vi "Release v1.0.vi"() -> ()   [LabVIEW 2014]
uses:
  <vilib>/Instr/_visa.llb/VISA Configure Serial Port (Instr).vi
  <vilib>/addons/control/pid/NI_PID_autopid.lvlib
panel:
  in  "Tab Control":T1(tab)
  in  "yaw PID gains":T2={"proportional gain (Kc)"=0.1, "integral time (Ti, min)"=0.001, "derivative time (Td, min)"=0.001} {"derivative time (Td, min)" step=0.001 format="%.3f"; "integral time (Ti, min)" step=0.01 format="%.3f"; "proportional gain (Kc)" step=0.1 format="%.3f"}
  in  "pitch PID gains":T2={"proportional gain (Kc)"=0.1, "integral time (Ti, min)"=0.001, "derivative time (Td, min)"=0.001} {"derivative time (Td, min)" step=0.001 format="%.3f"; "integral time (Ti, min)" step=0.01 format="%.3f"; "proportional gain (Kc)" step=0.1 format="%.3f"}
  in  "roll PID gains":T2={"proportional gain (Kc)"=0.1, "integral time (Ti, min)"=0.001, "derivative time (Td, min)"=0.001} {"derivative time (Td, min)" step=0.001 format="%.3f"; "integral time (Ti, min)" step=0.01 format="%.3f"; "proportional gain (Kc)" step=0.1 format="%.3f"}
  out "Celda 4":dbl
  out "Celda 3":dbl
  out "Celda 2":dbl
  out "Celda 1":dbl
  out "Celda 1":dbl(slide) scale=-1250.0..1250.0
  out "Celda 2":dbl(slide) scale=-1250.0..1250.0
  out "Celda 3":dbl(slide) scale=-1250.0..1250.0
  out "Celda 4":dbl(slide) scale=-1250.0..1250.0
  out "YAW PID":dbl
  out "yaw":cluster{"roll":dbl, "ROLL":dbl, dbl}(graph)
  out "yaw imu":dbl
  out "pitch imu":dbl
  out "PITCH PID":dbl
  out "PITCH":cluster{"roll":dbl, "ROLL":dbl, dbl}(graph)
  out "roll imu":dbl
  out "ROLL PID":dbl
  out "ROLL":cluster{"roll":dbl, "ROLL":dbl, dbl}(graph)
  out "Altura SENS":dbl
  in  "YAW":dbl(slide) scale=-25.0..25.0
  in  "PITCH 2":dbl(slide) caption="Roll" scale=-10.0..20.0
  in  "ROLL":dbl(slide) scale=-20.0..10.0
  in  "X":i64(slide) scale=-30.0..30.0
  in  "Y":i64(slide) scale=-30.0..30.0
  in  "?":i64(slide)=260 step=5 scale=220.0..290.0
  in  "PID ON?":bool
  out "bytes read":u32
  out "read string":string
  in  "stop":bool
  in  "baud rate":u32=115200
  in  "data bits":u16=8 min=5 max=8 step=1
  in  "parity":u16(ring) items=["None", "Odd", "Even", "Mark", "Space"]
  in  "stop bits":u16=10
  in  "flow control":u16
  in  "timeout (ms)":u32=10000
  in  "buffer size":u32=256
  in  "instr name":string="Arduino"
  in  "error in":errorcluster
  out "error out":errorcluster
  out "status":bool
  out "X 2":dbl
  out "Y 2":dbl
  out "Z":dbl
  in  "Stop":bool
  out "Write Buffer":string
  out "servo 2":dbl
  out "servo 4":dbl
  out "servo 5":dbl
  out "servo 6":dbl
  out "servo 1":dbl
  out "servo 3":dbl
  # "error"
  # "error"
  # "error"
  # "Z"
  # "el servo 1 responde al reves que los otros 5"
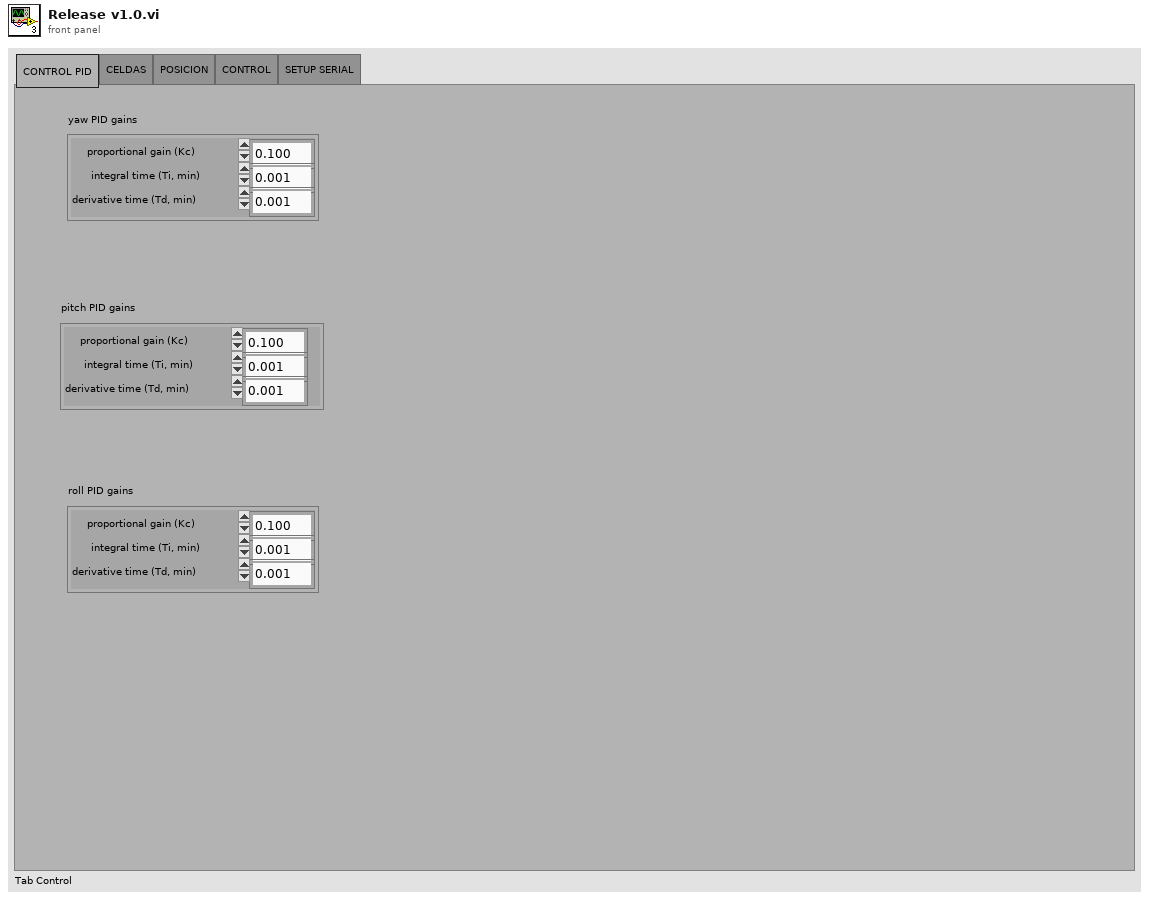
[diagram p1: front panel]
types:
  T1 = enum32{"CONTROL PID", "CELDAS", "POSICION", "CONTROL", "SETUP SERIAL"}
  T2 = cluster{"proportional gain (Kc)":dbl, "integral time (Ti, min)":dbl, "derivative time (Td, min)":dbl}
  T3 = cluster{"controller type":u16, "relay cycles":i32, "relay amplitude":dbl, "control specification":u16, "PV noise level":dbl}
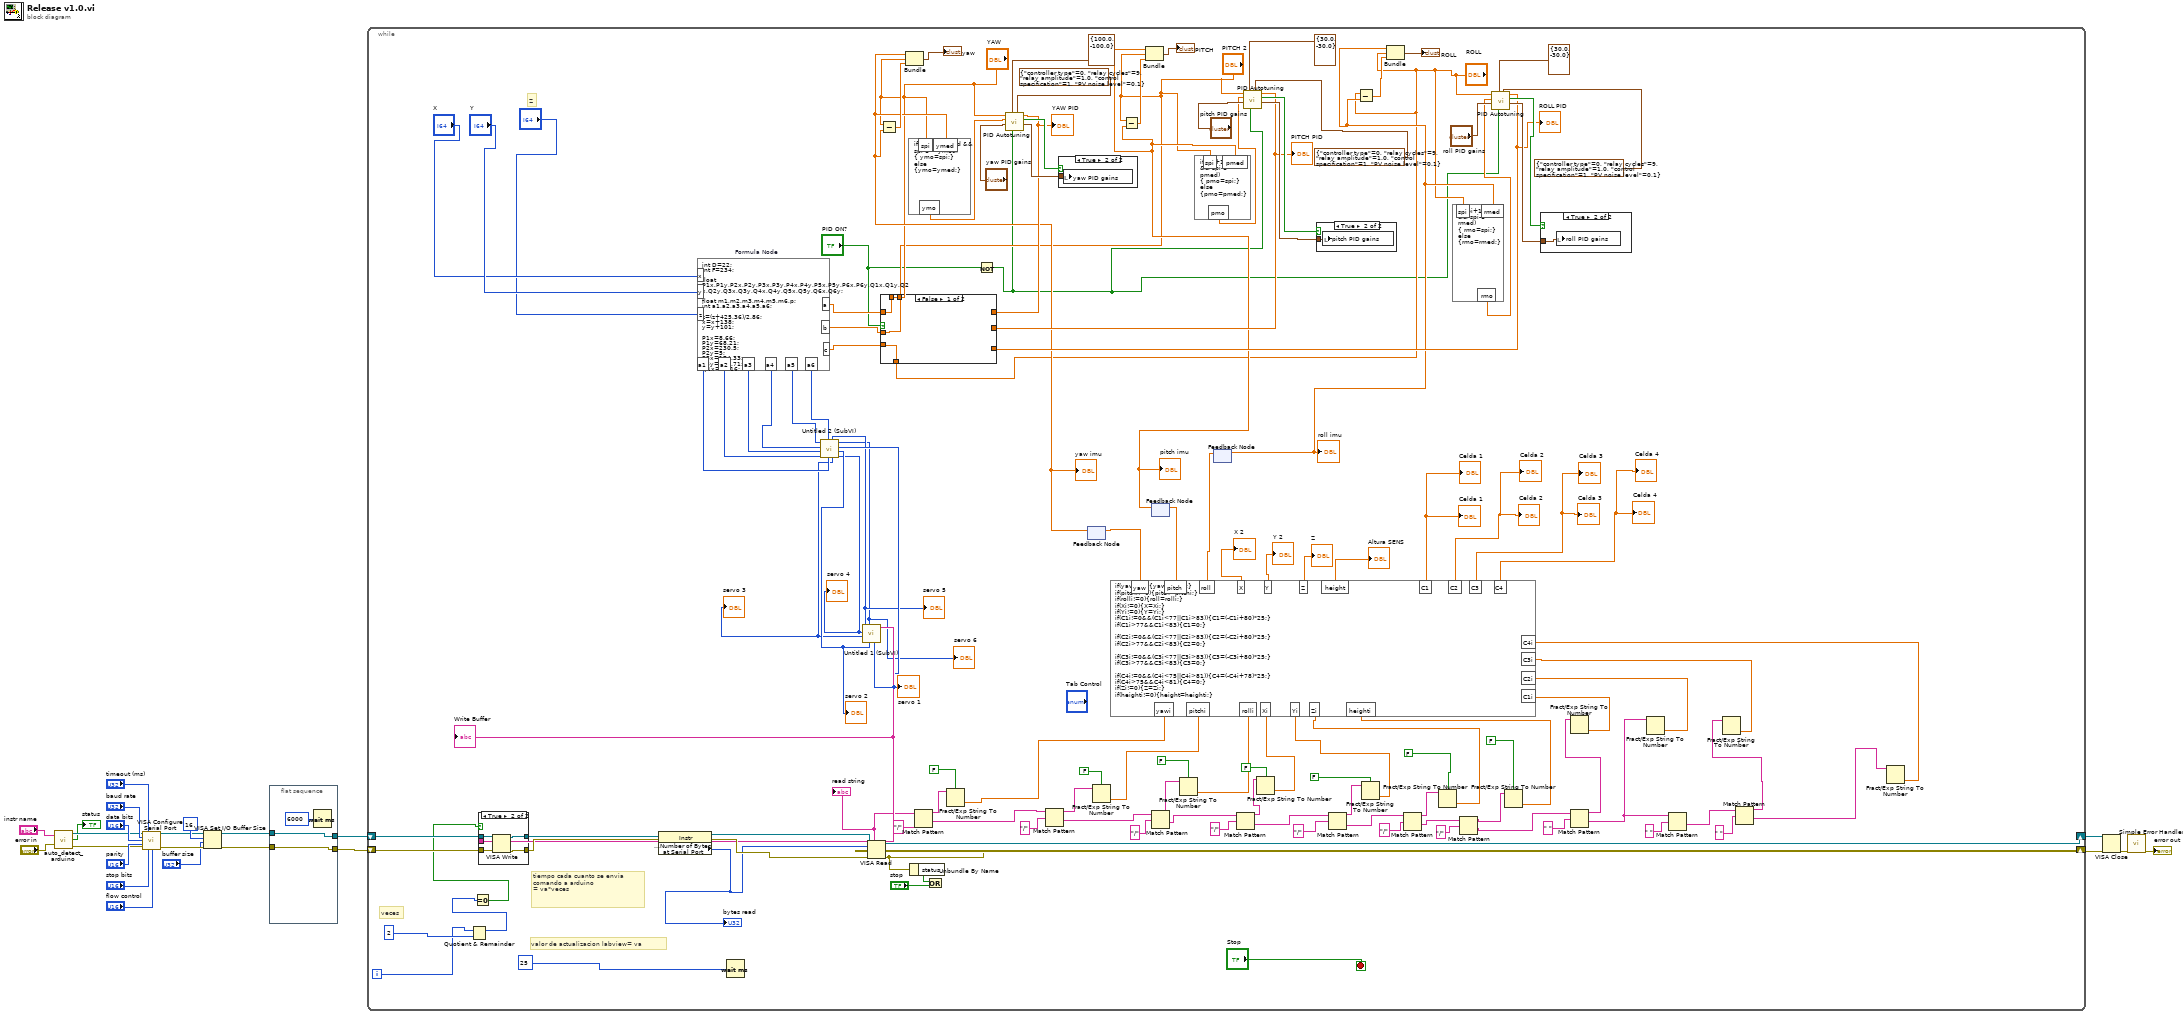
[diagram p0: block diagram]
diagram:
  n1 = call "auto_detect_arduino.vi"("instr name"="instr name", "error in"="error in") -> ("VISA resource name"=w16:refnum<visa-resource-name>, "status"=→"status":bool, "error out"=w15:errorcluster)
  n2 = call-poly "VISA Configure Serial Port"("VISA resource name"=w16, "timeout (10sec)"="timeout (ms)", "baud rate (9600)"="baud rate", "data bits (8)"="data bits", "parity (0:none)"="parity", "error in (no error)"=w15, "stop bits (10: 1 bit)"="stop bits", "flow control (0:none)"="flow control") -> ("VISA resource name out"=w12:refnum<visa-resource-name>, "error out"=w11:errorcluster)  [unwired: 6 in]
  n3 = VISA Set I/O Buffer Size(VISA resource name=w12, mask (16)=u16 16 ("I/O Receive\nBuffer mask"), size (4096)="buffer size", error in (no error)=w11) -> (VISA resource name out=w3:refnum<visa-resource-name>, error out=w1:errorcluster)
  n4 = flat-sequence {
    tunnel: [w25] -> w4
    tunnel: w3 -> [w25]
    tunnel: [w24] -> w2
    tunnel: w1 -> [w24]
    frame #0 {
      n5 = Wait (ms)(milliseconds to wait=u32 6000) -> ()  [unwired: 1 out]
    }
  }
  n6 = while {
    shift-right: [w133] -> w23
    shift-left: w4 -> [w156]
    shift-right: [w147] -> w5
    shift-left: w2 -> [w155]
    i -> [w144]
    stop <- "Stop" stop-if-true
    # "tiempo cada cuanto se envia\ncomando a arduino\n= va*veces"
    # "veces"
    # "valor de actualizacion labview= va"
    # "Z"
    n7 = Quotient & Remainder(x=w144, y=2) -> (x-y*floor(x/y)=w143:i32)  [unwired: 1 out]
    n8 = Equal To 0?(x=w143) -> (x = 0?=w142:bool)
    n9 = Wait (ms)(milliseconds to wait=u32 25) -> ()  [unwired: 1 out]
    n10 = Not(x="PID ON?") -> (.not. x?=w27:bool)
    n11 = feedback #1() -> (w63:dbl)  [unwired: 1 in]
    "yaw imu" <- w63
    n12 = Subtract(x="YAW", y=w63) -> (x-y=w82:dbl)
    n13 = Bundle("yaw"=w63, "YAW"="YAW", w82) -> (→"yaw":cluster{"yaw":dbl, "YAW":dbl, dbl})  [unwired: 1 in]
    n14 = formula code="if(spi+1>ymed && spi-1 < ymed)\n{ ymo=spi;}\nelse\n{ymo=ymed;}"("spi"="YAW", "ymed"=w63) -> ("ymo"=w58:dbl)
    n15 = call <vilib>:"PID Autotuning.vi"("autotuning parameters"=T3 {"controller type"=0, "relay cycles"=9, "relay amplitude"=1.0, "control specification"=1, "PV noise level"=0.1} ("autotuning initial parameters"), "reinitialize? (F)"=w27, "output range"=cluster{"output high":dbl, "output low":dbl} {"output high"=100.0, "output low"=-100.0}, "PID gains"="yaw PID gains", "process variable"=w58, "setpoint"="YAW") -> ("PID gains out"=w76:T2, "tuning completed?"=w77:bool, "output"=w68:dbl)  [unwired: 2 in, 1 out]
    "YAW PID" <- w68
    n16 = case shown="True" w77 {
      tunnel: w76 -> [_ w165]
      frame False {
      }
      frame True {
        n17 = local write "yaw PID gains"(w165) -> ()
      }
    }
    n18 = feedback #2() -> (w61:dbl)  [unwired: 1 in]
    "pitch imu" <- w61
    n19 = Subtract(x="PITCH 2", y=w61) -> (x-y=w86:dbl)
    n20 = Bundle("pitch"=w61, "PITCH 2"="PITCH 2", w86) -> (→"PITCH":cluster{"pitch":dbl, "PITCH 2":dbl, dbl})  [unwired: 1 in]
    n21 = formula code="if(spi+1>pmed && spi-1 < pmed)\n{ pmo=spi;}\nelse\n{pmo=pmed;}"("spi"="PITCH 2", "pmed"=w61) -> ("pmo"=w57:dbl)
    n22 = feedback #3() -> (w60:dbl)  [unwired: 1 in]
    "roll imu" <- w60
    n23 = call <vilib>:"PID Autotuning.vi"("autotuning parameters"=T3 {"controller type"=0, "relay cycles"=9, "relay amplitude"=1.0, "control specification"=1, "PV noise level"=0.1} ("autotuning initial parameters"), "reinitialize? (F)"=w27, "output range"=cluster{"output high":dbl, "output low":dbl} {"output high"=30.0, "output low"=-30.0}, "PID gains"="pitch PID gains", "process variable"=w57, "setpoint"="PITCH 2") -> ("PID gains out"=w73:T2, "tuning completed?"=w74:bool, "output"=w66:dbl)  [unwired: 2 in, 1 out]
    "PITCH PID" <- w66
    n24 = case shown="True" w74 {
      tunnel: w73 -> [_ w164]
      frame False {
      }
      frame True {
        n25 = local write "pitch PID gains"(w164) -> ()
      }
    }
    n26 = Subtract(x="ROLL", y=w60) -> (x-y=w87:dbl)
    n27 = Bundle("roll"=w60, "ROLL"="ROLL", w87) -> (→"ROLL":cluster{"roll":dbl, "ROLL\n":dbl, dbl})  [unwired: 1 in]
    n28 = formula code="if(spi+1>rmed && spi-1 < rmed)\n{ rmo=spi;}\nelse\n{rmo=rmed;}"("spi"="ROLL", "rmed"=w60) -> ("rmo"=w55:dbl)
    n29 = call <vilib>:"PID Autotuning.vi"("autotuning parameters"=T3 {"controller type"=0, "relay cycles"=9, "relay amplitude"=1.0, "control specification"=1, "PV noise level"=0.1} ("autotuning initial parameters"), "reinitialize? (F)"=w27, "output range"=cluster{"output high":dbl, "output low":dbl} {"output high"=30.0, "output low"=-30.0}, "PID gains"="roll PID gains", "process variable"=w55, "setpoint"="ROLL") -> ("PID gains out"=w70:T2, "tuning completed?"=w71:bool, "output"=w64:dbl)  [unwired: 2 in, 1 out]
    "ROLL PID" <- w64
    n30 = case shown="False" "PID ON?" {
      tunnel: [w159 w162] -> w69
      tunnel: w68 -> [_ w162]
      tunnel: [w158 w161] -> w67
      tunnel: w66 -> [_ w161]
      tunnel: [w157 w160] -> w65
      tunnel: w64 -> [_ w160]
      tunnel: "YAW" -> [w159 _]
      tunnel: "PITCH 2" -> [w158 _]
      tunnel: "ROLL" -> [w157 _]
      frame False {
      }
      frame True {
      }
    }
    n31 = formula code="int D=22;\nint F=234;\n\nfloat P1x,P1y,P2x,P2y,P3x,P3y,P4x,P4y,P5x,P5y,P6x,P6y,Q1x,Q1y,Q2x,Q2y,Q3x,Q3y,Q4x,Q4y,Q5x,Q5y,Q6x,Q6y;\n\nfloat m1,m2,m3,m4,m5,m6,p;\nint a1,a2,a3,a4,a5,a6;\n\nz=(z+425.36)/2.86;\nx=x+138;\ny=y+101;\n\nP1x=8.66;\nP1y=68.21;\nP2x=230.5;\nP2y=5;\nP3x=174.33;\nP3y=233.71;\nQ1x=45.16;\nQ1y=5;\nQ2x=267;\nQ2y=68.21;\nQ3x=101.33;\nQ3y=233.71;\n\n\nP4x=-81.5;\nP4y=-38.4;\nP5x=74;\nP5y=-51.3;\nP6x=7.5;\nP6y=89.8;\nQ4x=-74;\nQ4y=-51.3;\nQ5x=81.5;\nQ5y=-38.4;\nQ6x=-7.5;\nQ6y=89.8;\n\n\n//yaw\na=-a/57.3;\n\n//pitch\nb=b/57.3;\n\n//roll\nc=c/57.3;\n\n\nm1= sqrt((Q4x*(cos(c)*cos(a)+sin(a)*sin(b)*sin(c))+Q4y*(cos(a)*sin(b)*sin(c)-sin(a)*cos(c))+x-Q1x)**2+(Q4x*sin(a)*cos(b)+Q4y*cos(a)*cos(b)+y-Q1y)**2+(Q4x*(sin(a)*sin(b)*cos(c)-cos(a)*sin(c))+Q4y*(sin(a)*sin(c)+cos(a)*sin(b)*cos(c))+z)**2);\nm2= sqrt((P5x*(cos(c)*cos(a) +sin(a)*sin(b)*sin(c))+ P5y*(cos(a)*sin(b)*sin(c)-sin(a)*cos(c))+x-P2x)**2+(P5x*sin(a)*cos(b) +P5y*cos(a)*cos(b) +y-P2y)**2+(P5x*(sin(a)*sin(b)*cos(c)-cos(a)*sin(c)) +P5y*(sin(a)*sin(c) +cos(a)*sin(b)*cos(c))+z)**2);\nm3= sqrt((Q5x*(cos(c)*cos(a)+sin(a)*sin(b)*sin(c))+Q5y*(cos(a)*sin(b)*sin(c)-sin(a)*cos(c))+x-Q2x)**2+(Q5x*sin(a)*cos(b)+Q5y*cos(a)*cos(b)+y-Q2y)**2+(Q5x*(sin(a)*sin(b)*cos(c)-cos(a)*sin(c))+Q5y*(sin(a)*sin(c)+cos(a)*sin(b)*cos(c))+z)**2);\nm4= sqrt((P6x*(cos(c)*cos(a)+sin(a)*sin(b)*sin(c))+ P6y*(cos(a)*sin(b)*sin(c)-sin(a)*cos(c))+x-P3x)**2 +(P6x*sin(a)*cos(b) +P6y*cos(a)*cos(b) +y-P3y)**2 +(P6x*(sin(a)*sin(b)*cos(c)-cos(a)*sin(c))+P6y*(sin(a)*sin(c) +cos(a)*sin(b)*cos(c))+z)**2);\nm5= sqrt((Q6x*(cos(c)*cos(a)+sin(a)*sin(b)*sin(c))+Q6y*(cos(a)*sin(b)*sin(c)-sin(a)*cos(c))+x-Q3x)**2+(Q6x*sin(a)*cos(b)+Q6y*cos(a)*cos(b)+y-Q3y)**2+(Q6x*(sin(a)*sin(b)*cos(c)-cos(a)*sin(c))+Q6y*(sin(a)*sin(c)+cos(a)*sin(b)*cos(c))+z)**2);\nm6= sqrt((P4x*(cos(c)*cos(a)+sin(a)*sin(b)*sin(c))+ P4y*(cos(a)*sin(b)*sin(c)-sin(a)*cos(c))+x-P1x)**2 +(P4x*sin(a)*cos(b) +P4y*cos(a)*cos(b) +y-P1y)**2 +(P4x*(sin(a)*sin(b)*cos(c)-cos(a)*sin(c))+P4y*(sin(a)*sin(c) +cos(a)*sin(b)*cos(c))+z)**2);\n\n\n\n\n\n\n\na1=floor(180-(acos(((-D**4)+(2*(D**2)*(F**2))+(2*(D**2)*(m1**2))-(F**4)+(2*(F**2)*(m1**2))-(m1**4))**(1/2)/(2*D*m1)))*180/3.1416);\na2=floor(180-(acos(((-D**4)+(2*(D**2)*(F**2))+(2*(D**2)*(m2**2))-(F**4)+(2*(F**2)*(m2**2))-(m2**4))**(1/2)/(2*D*m2)))*180/3.1416);\na3=floor((acos(((-D**4)+(2*(D**2)*(F**2))+(2*(D**2)*(m3**2))-(F**4)+(2*(F**2)*(m3**2))-(m3**4))**(1/2)/(2*D*m3)))*180/3.1416);\n//motor 4 es el nuevo fallado\na4=floor((acos(((-D**4)+(2*(D**2)*(F**2))+(2*(D**2)*(m4**2))-(F**4)+(2*(F**2)*(m4**2))-(m4**4))**(1/2)/(2*D*m4)))*180/3.1416);\na5=floor((acos(((-D**4)+(2*(D**2)*(F**2))+(2*(D**2)*(m5**2))-(F**4)+(2*(F**2)*(m5**2))-(m5**4))**(1/2)/(2*D*m5)))*180/3.1416);\na6=floor(180-(acos(((-D**4)+(2*(D**2)*(F**2))+(2*(D**2)*(m6**2))-(F**4)+(2*(F**2)*(m6**2))-(m6**4))**(1/2)/(2*D*m6)))*180/3.1416);"("x"="X", "y"="Y", "z"="?", "a"=w69, "b"=w67, "c"=w65) -> ("a1"=w141:i32, "a2"=w138:i32, "a3"=w140:i32, "a4"=w137:i32, "a5"=w139:i32, "a6"=w136:i32)
    n32 = call "Untitled 2 (SubVI).vi"("Numeric 12"=w141, "Numeric 7"=w136, "Numeric 9"=w138, "Numeric 11"=w140, "Numeric 8"=w137, "Numeric 10"=w139) -> ("Numeric 2"=w128:u8, "Numeric 5"=w131:u8, "Numeric 6"=w132:u8, "Numeric"=w127:u8, "Numeric 4"=w130:u8, "Numeric 3"=w129:u8)
    "servo 6" <- w127
    "servo 5" <- w129
    "servo 4" <- w128
    "servo 2" <- w131
    "servo 1" <- w132
    "servo 3" <- w130
    n33 = call "Untitled 1 (SubVI).vi"("Numeric"=w132, "Numeric 2"=w131, "Numeric 6"=w127, "Numeric 3"=w130, "Numeric 4"=w128, "Numeric 5"=w129) -> ("String"=w134:string)  [unwired: 5 in]
    "Write Buffer" <- w134
    n34 = case shown="True" w142 {
      tunnel: w156 -> [w167 w172]
      tunnel: w155 -> [w166 w171]
      tunnel: [w167 w170] -> w149
      tunnel: [w166 w169] -> w148
      tunnel: w134 -> [_ w168]
      frame False {
      }
      frame True {
        n35 = VISA Write(VISA resource name=w172, write buffer=w168, error in (no error)=w171) -> (VISA resource name out=w170:refnum<visa-resource-name>, error out=w169:errorcluster)  [unwired: 1 out]
      }
    }
    n36 = property class="Instr"(reference=w149, error in=w148) -> (reference out=w151:refnum<visa-resource-name>, error out=w150:errorcluster, "Serial Settings:Number of Bytes at Serial Port"=w135:u32)
    "bytes read" <- w135
    n37 = VISA Read(VISA resource name=w151, byte count=w135, error in (no error)=w150) -> (VISA resource name out=w133:refnum<visa-resource-name>, read buffer=w117:string, error out=w147:errorcluster)  [unwired: 1 out]
    "read string" <- w117
    n38 = Unbundle By Name(w147) -> ("status"=w120:bool)
    n39 = Match Pattern(string=w117, regular expression="/") -> (before substring=w118:string, after substring=w125:string)  [unwired: 1 in, 2 out]
    n40 = Or(x=w120, y="stop") -> ()  [unwired: 1 out]
    n41 = Fract/Exp String To Number(use system decimal point (T)=FALSE, string=w118) -> (number=w102:dbl)  [unwired: 2 in, 1 out]
    n42 = Match Pattern(string=w125, regular expression="/") -> (before substring=w123:string, after substring=w115:string)  [unwired: 1 in, 2 out]
    n43 = Fract/Exp String To Number(use system decimal point (T)=FALSE, string=w123) -> (number=w103:dbl)  [unwired: 2 in, 1 out]
    n44 = Match Pattern(string=w115, regular expression="/") -> (before substring=w114:string, after substring=w112:string)  [unwired: 1 in, 2 out]
    n45 = Fract/Exp String To Number(use system decimal point (T)=FALSE, string=w114) -> (number=w101:dbl)  [unwired: 2 in, 1 out]
    n46 = Match Pattern(string=w112, regular expression="/") -> (before substring=w109:string, after substring=w107:string)  [unwired: 1 in, 2 out]
    n47 = Fract/Exp String To Number(use system decimal point (T)=FALSE, string=w109) -> (number=w100:dbl)  [unwired: 2 in, 1 out]
    n48 = Match Pattern(string=w107, regular expression="/") -> (before substring=w105:string, after substring=w94:string)  [unwired: 1 in, 2 out]
    n49 = Fract/Exp String To Number(use system decimal point (T)=FALSE, string=w105) -> (number=w99:dbl)  [unwired: 2 in, 1 out]
    n50 = Match Pattern(string=w94, regular expression="/") -> (before substring=w92:string, after substring=w50:string)  [unwired: 1 in, 2 out]
    n51 = Fract/Exp String To Number(use system decimal point (T)=FALSE, string=w92) -> (number=w98:dbl)  [unwired: 2 in, 1 out]
    n52 = Match Pattern(string=w50, regular expression="/") -> (before substring=w48:string, after substring=w47:string)  [unwired: 1 in, 2 out]
    n53 = Fract/Exp String To Number(use system decimal point (T)=FALSE, string=w48) -> (number=w91:dbl)  [unwired: 2 in, 1 out]
    n54 = case shown="True" w71 {
      tunnel: w70 -> [_ w163]
      frame False {
      }
      frame True {
        n55 = local write "roll PID gains"(w163) -> ()
      }
    }
    n56 = Match Pattern(string=w47, regular expression=" ") -> (before substring=w52:string, after substring=w42:string)  [unwired: 1 in, 2 out]
    n57 = Fract/Exp String To Number(string=w52) -> (number=w37:dbl)  [unwired: 3 in, 1 out]
    n58 = Fract/Exp String To Number(string=w42) -> (number=w36:dbl)  [unwired: 3 in, 1 out]
    n59 = Match Pattern(string=w42, regular expression=" ") -> (after substring=w44:string)  [unwired: 1 in, 3 out]
    n60 = Match Pattern(string=w44, regular expression=" ") -> (before substring=w43:string, after substring=w45:string)  [unwired: 1 in, 2 out]
    n61 = Fract/Exp String To Number(string=w43) -> (number=w34:dbl)  [unwired: 3 in, 1 out]
    n62 = Fract/Exp String To Number(string=w45) -> (number=w33:dbl)  [unwired: 3 in, 1 out]
    n63 = formula code="if(yawi!=0){yaw=yawi;}\nif(pitchi!=0){pitch=pitchi;}\nif(rolli!=0){roll=rolli;}\nif(Xi!=0){X=Xi;}\nif(Yi!=0){Y=Yi;}\nif(C1i!=0&&(C1i<77||C1i>83)){C1=(-C1i+80)*25;}\nif(C1i>77&&C1i<83){C1=0;}\n\nif(C2i!=0&&(C2i<77||C2i>83)){C2=(-C2i+80)*25;}\nif(C2i>77&&C2i<83){C2=0;}\n\nif(C3i!=0&&(C3i<77||C3i>83)){C3=(-C3i+80)*25;}\nif(C3i>77&&C3i<83){C3=0;}\n\nif(C4i!=0&&(C4i<75||C4i>81)){C4=(-C4i+78)*25;}\nif(C4i>75&&C4i<81){C4=0;}\nif(Zi!=0){Z=Zi;}\nif(heighti!=0){height=heighti;}"("yawi"=w102, "Zi"=w98, "pitchi"=w103, "rolli"=w101, "Yi"=w99, "Xi"=w100, "heighti"=w91, "C1i"=w37, "C2i"=w36, "C3i"=w34, "C4i"=w33) -> ("yaw"=w95:dbl, "pitch"=w97:dbl, "roll"=w96:dbl, "X"=→"X 2":dbl, "Y"=→"Y 2":dbl, "Z"=→"Z":dbl, "height"=→"Altura SENS":dbl, "C1"=→"Celda 1" →"Celda 1":dbl, "C2"=→"Celda 2" →"Celda 2":dbl, "C3"=→"Celda 3" →"Celda 3":dbl, "C4"=→"Celda 4" →"Celda 4":dbl)
    n64 = feedback-in #1(w95) -> ()
    n65 = feedback-in #2(w97) -> ()
    n66 = feedback-in #3(w96) -> ()
  }
  n67 = VISA Close(VISA resource name=w23, error in (no error)=w5) -> (error out=w8:errorcluster)
  n68 = call <vilib>:"Simple Error Handler.vi"("error in (no error)"=w8) -> ("error out"=→"error out":errorcluster)  [unwired: 4 in, 4 out]
